vi "折叠行.vi"(8 "错误输入（无错误）":errorcluster, 9 "簇":cluster{"背景":u32, "前景":u32}={"背景"=16448250, "前景"=16448250}, 11 "引用":refnum<k24>) -> (0 "错误输出":errorcluster, 3 "Scintilla":refnum<k24>)   [LabVIEW 2018]
uses:
  ScintillaNET.dll
  System.Drawing
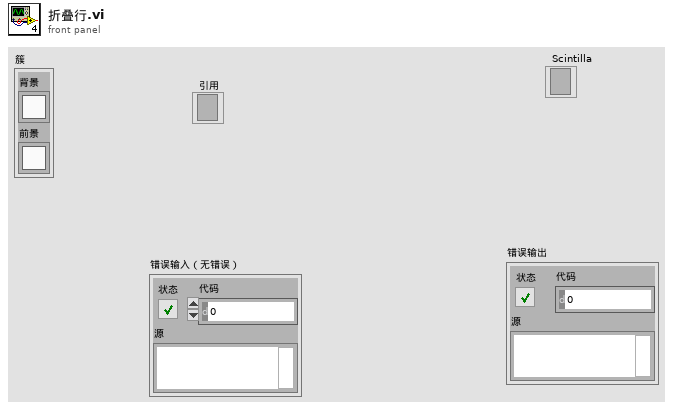
[diagram p1: front panel]
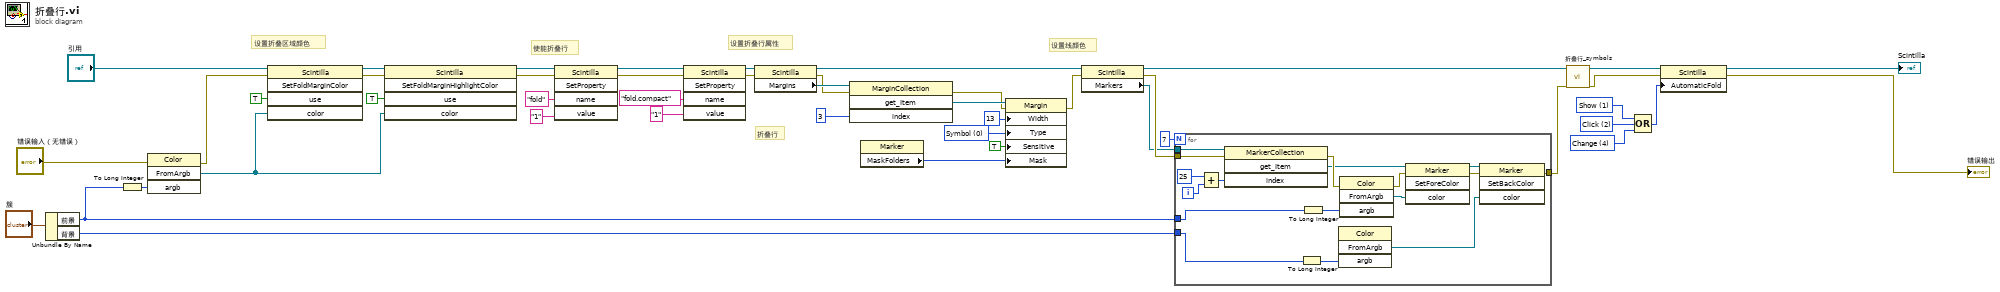
[diagram p0: block diagram]
diagram:
  w8 = 4 items=["None"=0, "Show"=1, "Click"=2, "Change"=4] ("AutomaticFold")
  w9 = 2 items=["None"=0, "Show"=1, "Click"=2, "Change"=4] ("AutomaticFold")
  w10 = 1 items=["None"=0, "Show"=1, "Click"=2, "Change"=4] ("AutomaticFold")
  w40 = 0 items=["Symbol", "Number", "BackColor", "ForeColor", "Text", "RightText", "Color"] ("Type")
  # "设置线颜色"
  # "使能折叠行"
  # "折叠行"
  # "设置折叠行属性"
  # "设置折叠区域颜色"
  n1 = Unbundle By Name("簇") -> ("前景"=w2:u32, "背景"=w1:u32)
  n2 = To Long Integer(number=w2) -> (32bit integer=w45:i32)
  n3 = invoke class="Color" method="FromArgb"(error in="错误输入（无错误）", "argb"=w45) -> (error out=w32:errorcluster, "FromArgb"=w42:refnum<k24>)  [unwired: 2 in, 2 out]
  n4 = invoke class="Scintilla" method="SetFoldMarginColor"(reference="引用", error in=w32, "use"=TRUE, "color"=w42) -> (reference out=w44:refnum<k24>, error out=w31:errorcluster)  [unwired: 1 in, 3 out]
  n5 = invoke class="Scintilla" method="SetFoldMarginHighlightColor"(reference=w44, error in=w31, "use"=TRUE, "color"=w42) -> (reference out=w35:refnum<k24>, error out=w27:errorcluster)  [unwired: 1 in, 3 out]
  n6 = invoke on="调用节点" class="Scintilla" method="SetProperty"(reference=w35, error in=w27, "name"="fold", "value"="1") -> (reference out=w24:refnum<k24>, error out=w23:errorcluster)  [unwired: 1 in, 3 out]
  n7 = invoke on="调用节点" class="Scintilla" method="SetProperty"(reference=w24, error in=w23, "name"="fold.compact", "value"="1") -> (reference out=w22:refnum<k24>, error out=w21:errorcluster)  [unwired: 1 in, 3 out]
  n8 = property class="Scintilla"(reference=w22, error in=w21) -> (reference out=w28:refnum<k24>, error out=w30:errorcluster, "Margins"=w36:refnum<k24>)
  n9 = invoke class="MarginCollection" method="get_Item"(reference=w36, error in=w30, "index"=3) -> (error out=w29:errorcluster, "get_Item"=w38:refnum<k24>)  [unwired: 1 in, 2 out]
  n10 = property on="属性节点" class="Marker"() -> ("MaskFolders"=w4:u32)  [unwired: 2 in, 2 out]
  n11 = property class="Margin"(reference=w38, error in=w29, "Width"=13, "Type"=w40, "Sensitive"=TRUE, "Mask"=w4) -> (error out=w17:errorcluster)  [unwired: 1 out]
  n12 = property on="属性节点" class="Scintilla"(reference=w28, error in=w17) -> (reference out=w13:refnum<k24>, error out=w16:errorcluster, "Markers"=w15:refnum<k24>)
  n13 = for {
    N: 7 -> [_]
    tunnel: w15 -> [w63]
    tunnel: w16 -> [w55]
    tunnel: [w52] -> w14
    tunnel: w2 -> [w48]
    tunnel: w1 -> [w47]
    i -> [w58]
    n14 = Add(x=25, y=w58) -> (x+y=w56:i32)
    n15 = invoke class="MarkerCollection" method="get_Item"(reference=w63, error in=w55, "index"=w56) -> (error out=w54:errorcluster, "get_Item"=w51:refnum<k24>)  [unwired: 1 in, 2 out]
    n16 = To Long Integer(number=w47) -> (32bit integer=w50:i32)
    n17 = To Long Integer(number=w48) -> (32bit integer=w60:i32)
    n18 = invoke class="Color" method="FromArgb"("argb"=w50) -> ("FromArgb"=w49:refnum<k24>)  [unwired: 3 in, 3 out]
    n19 = invoke class="Color" method="FromArgb"(error in=w54, "argb"=w60) -> (error out=w53:errorcluster, "FromArgb"=w59:refnum<k24>)  [unwired: 2 in, 2 out]
    n20 = invoke class="Marker" method="SetForeColor"(reference=w51, error in=w53, "color"=w59) -> (reference out=w62:refnum<k24>, error out=w61:errorcluster)  [unwired: 1 in, 2 out]
    n21 = invoke class="Marker" method="SetBackColor"(reference=w62, error in=w61, "color"=w49) -> (error out=w52:errorcluster)  [unwired: 1 in, 3 out]
  }
  n22 = call "折叠行_symbols.vi"("错误输入（无错误）"=w14, "引用"=w13) -> ("错误输出"=w6:errorcluster, "引用输出"=w12:refnum<k24>)  [unwired: 8 in]
  n23 = Compound Arithmetic op=OR(w10, w9, w8) -> (w7:i32)
  n24 = property on="属性节点" class="Scintilla"(reference=w12, error in=w6, "AutomaticFold"=w7) -> (reference out=→"Scintilla":refnum<k24>, error out=→"错误输出":errorcluster)
